vi "Encoder Buffer Updated.vi"(8 "error in (no error)":errorcluster, 10 "Encoder Positions":dbl[](array[numeric]), 11 "Business Logic in":refnum<class "Business Logic.lvclass">) -> (0 "error out":errorcluster, 3 "Business Logic out":refnum<class "Business Logic.lvclass">)   [LabVIEW 2025, in "Business Logic.lvlib" / "Business Logic.lvclass"]
uses:
  Business Logic.lvclass
  Business Logic.lvclass/Business Logic.ctl
  User Interface Messages/Update Graph Msg/Update Graph Msg.lvclass
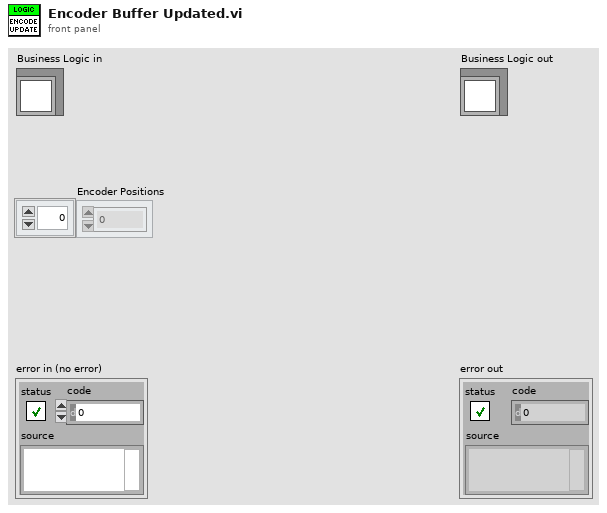
[diagram p1: front panel]
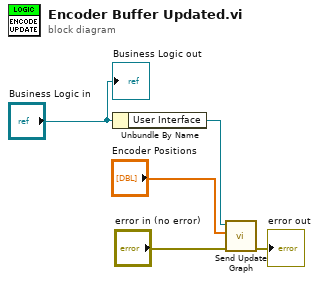
[diagram p0: block diagram]
diagram:
  n1 = Unbundle By Name("Business Logic in") -> ("User Interface"=w4:refnum<class "Message Enqueuer.lvclass">)
  n2 = call "Send Update Graph.vi"("error in (no error)"="error in (no error)", "Graph Data"="Encoder Positions", "Message Enqueuer"=w4) -> ("error out"=→"error out":errorcluster)  [unwired: 7 in, 1 out]
  "Business Logic out" <- "Business Logic in"
